vi "bangBangVelocityPlanning.vi"(0 "Game":refnum<class "Game.lvclass">, 5 "Robot in":refnum<class "Robot.lvclass">, 9 "Dest_array":T5(array[cluster]), 11 "type_of_use":T1, 12 "robots_test":T2[](array[typedef]), 13 "start":bool=TRUE) -> (4 "Robot out":refnum<class "Robot.lvclass">, 6 "replace":bool, 8 "velocityPlanningState":T3={"est_vel"=0.0, "dist_to_(Dest/L)"=0.0, "V0_model"=0.0, "max_dist_to_break"=0.0, "v_sent"=0.0, "traj_state"=enum."replace"})   [LabVIEW 2023, in "Game.lvclass"]
uses:
  Game.lvclass
  Robot_class/Robot.lvclass
  C:/Users/lucio/Desktop/roboime/SSL_AI/Object_class/Object.lvclass
  VelocityPlanningTest/Controls/velocityPlanningState.ctl
  VelocityPlanningTest/Controls/trajectoryState.ctl
  Communication_class/Paths/grSim Packet Command UDP Test Folder/grSim/grSim RobotReplacement.ctl
  Controls/typeOfUse.ctl
  Team_class/KeeperPlay.ctl
  Team_class/OffensivePlay.ctl
  Robot_class/Robot.lvclass/Robot.ctl
  Object_class/Object.lvclass/Object.ctl
  Game.lvclass/Game.ctl
  Team_class/Team.lvclass/Team.ctl
  Parameters_class/Parameters.lvclass/Parameters.ctl
  Robot_class/Read path_smooth.vi
  Object_class/Read x.vi
  Object_class/Read y.vi
  Robot_class/Write v_tang.vi
  Robot_class/Write v_norm.vi
  Robot_class/Write v_ang.vi
  Robot_class/Write est_v_norm.vi
  Robot_class/Write est_v_tang.vi
  <vilib>/Analysis/_algsub.llb/Real Vector Norm.vi
  Robot_class/Read orientation.vi
  Read OffensiveTeam.vi
  Read FieldRef.vi
  Read KeeperTeam.vi
  Read NewParameters.vi
  Read Parameters.lvclass.vi
  Parameters_class/Read PID gains Vel_desired.vi
  Parameters_class/Read StopVelocity.vi
  Parameters_class/Read Debug.vi
  Parameters_class/Read PID gains Angle.vi
  Parameters_class/Read PID gains Angle To Turn.vi
  Parameters_class/Read MaxOutputAngle.vi
  Parameters_class/Read bangBangParameters.vi
  Parameters_class/Read Enviroment.vi
  Parameters_class/Read PID per ID.vi
  Team_class/Read KeeperPlay.vi
  Team_class/Read OffensivePlay.vi
  Robot_class/Read robotKickState.vi
  Robot_class/Read dest_x.vi
  Robot_class/Read dest_y.vi
  Robot_class/Read v_tang.vi
  Robot_class/Read v_norm.vi
  Object_class/Read position(x,y).vi
  Ally_class/Ally.lvclass
  C:/Users/lucio/Desktop/roboime/SSL_AI/Team_class/Team.lvclass
  Field_class/Field.lvclass
  Parameters_class/Parameters.lvclass
  Utilities_class/Utilities.lvclass
  <vilib>/Analysis/NI_AALPro.lvlib
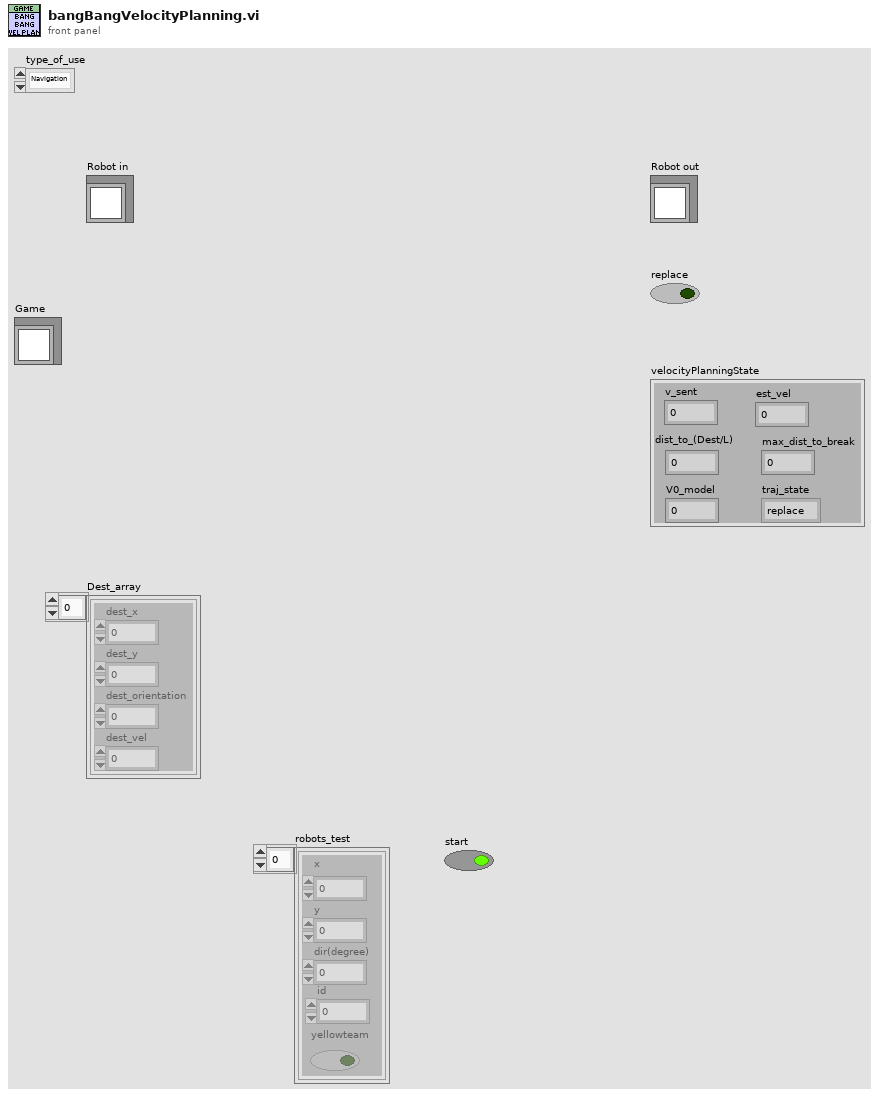
[diagram p1: front panel]
types:
  T1 = typedef "typeOfUse.ctl" = enum16{"Navigation", "ZigZag", "grSimTest"}
  T2 = typedef "grSim RobotReplacement.ctl" = cluster{"x":dbl, "y":dbl, "dir(degree)":dbl, "yellowteam":bool, "id":u32}
  T3 = typedef "velocityPlanningState.ctl" = cluster{"est_vel":dbl, "dist_to_(Dest/L)":dbl, "V0_model":dbl, "max_dist_to_break":dbl, "v_sent":dbl, "traj_state":T4}
  T4 = typedef "trajectoryState.ctl" = enum16{"stop", "replace", "circle", "line"}
  T5 = cluster{"dest_x":dbl, "dest_y":dbl, "dest_orientation":dbl, "dest_vel":dbl}[]
  T6 = typedef "OffensivePlay.ctl" = enum16{"5RobotsPassGamePlay", "5PreparePassGame", "5RobotsKeeperGame", "KeeperPassToStriker", "5RobotsNormalGamePlay", "PrepareKeeperPass", "ACBPass", "ABCPass", "PrepareTriplePass", "TableWithStriker", "TableWith2ndStrikerPlay", "PrepareDoublePass", "PrepareRollToPass", "SimplePass", "PreparePass", "PassToStriker", "BallOutOfField", "PassTo2ndStriker", "StopOffensive", "Prepare Penalty Enemy", "EnemyPossessionAtEnemyField", "EnemyPossesionAtOurField", "TestPlay", "PreparePenaltyAlly", "KickPenaltyAlly", "PrepareKickoffAlly", "PrepareKickoffEnemy", "IndirectEnemy", "DirectEnemy", "PreparePassInGame1", "NormalGame", "DirectKick", "Pass", "Halt", "Timeout", "PassPlay", "PenaltyEnemy"}
  T7 = typedef "KeeperPlay.ctl" = enum16{"SimpleBallPlacementAlly", "BallPlacementAlly", "BallPlacementEnemy", "ZigZag", "Goto", "NormalGame", "KeeperPlay", "Halt", "Timeout", "PenaltyEnemy", "TestPlay"}
  T8 = typedef "NewParameters.ctl" = cluster{"PenaltyDistance":dbl, "DistanceAttackerToBackBall":dbl, "Division":enum16{"Div B", "Div A"}, "DistanceToAvoidyEnemyRobot":dbl, "BallPlacementDistance":dbl, "DisatanceBehindBallToStealBall":dbl, "MaxDistanceToPositionKickoff":dbl, "BlockEnemyTarget":bool, "MaxStopVAng":dbl, "DistanceMarkerToEnemy":dbl, "IgnoreDribblerContact":bool, "DistanceToBeginEnemyPosession":dbl, "GoToBallWhenEnemyNotMoving":bool, "EnemyDistanceToReduceVelocity":dbl, "TurnOnEnemyDistanceToReduceVelocity":bool, "EnemyDistanceToShootOutBall":dbl, "DefenseKickBall":bool, "MoreKickToGoal? (0-0.3)":dbl, "ChipKickInEnemyField":bool, "ShootOutRobotId":dbl, "FieldLenghtDenominatorInShootOut":dbl, "AdjustPositionInBallPlacement":bool, "PowerGodPass":dbl, "VelocityAbortEnemyPos":dbl, "MaxDistToBeginPass":dbl, "MinDistToBeginPass":dbl, "VelocityInDirects":dbl, "BadDribblerIDs":i32[], "NewKickToDistanceAroundBall":dbl, "PowerAvoidColisionMarker":dbl, "DistanceToAvoidColisionMarker":dbl, "AvoidBallKick":dbl, "DistanceTryKick":dbl, "SuicideKickDIstance":dbl, "AdjustFirstKickDistance":dbl, "AvoidAimLessKick":dbl, "DistanceToAvoidyEnemyShootRobot ":dbl, "NumberOfMarkers":dbl, "PotField":bool, "PIDLateral":bool, "MinDistanceFirstKickX":dbl, "MinDistanceFirstKickY":dbl, "FractionOfDistToTouchGround\nAfterChipKick":dbl, "FractionOfKickxWhen\nComposedWithKickz":dbl, "Style":T9, "MoveInTurnState":bool, "DistFromEnemyToConsider\nMoveInTurnState":dbl, "CascadePID":bool, "TurnAroundParameters":cluster{"Radius":dbl, "Multiplier":dbl, "ChordAngle":dbl}, "SafeDriveVel":dbl, "DistanceToGoToBackBall":dbl, "minDistanceToNotFinishEnemyPossession":dbl, "OneTouchShot":cluster{"angleFactor":dbl, "maxAngle":dbl, "Attack":bool, "Defense":bool}, "OpenAngleToGoal":cluster{"minAngle":dbl, "maxAngle":dbl, "minEvaluation":dbl}, "ShotInterception":cluster{"shotSpeed":dbl, "minEnemySpeed":dbl, "maxEnemySpeed":dbl, "minEvaluation":dbl}, "AllyTeamArray":T10[], "maxDefendersNumber":i32, "Zone":cluster{"GuardPositionArray":dbl[][], "ZoneMidField":dbl[], "CenterForwardWidth":dbl}, "MinEvaluationToShoot":dbl, "PassInterception":cluster{"maxPassSpeed":dbl, "minPassSpeed":dbl, "minEnemySpeed":dbl, "chipPassDistance":dbl, "chipPassEvaluation":dbl, "minEvaluation":dbl, "maxEnemySpeed":dbl}, "PassDistance":cluster{"maxDistance":dbl, "minDistance":dbl}, "receiverSpeed":dbl, "maxBallSpeed":dbl, "slackTime":dbl}
  T9 = typedef "Style.ctl" = enum16{"Insanity", "Offensive", "Defensive"}
  T10 = typedef "AllyTeam.ctl" = enum16{"Keeper", "Defender", "Attacker"}
  T11 = cluster{"(Kc)":dbl, "(Ti, min)":dbl, "(Td, min)":dbl}
  T12 = typedef "bangBangControlParameters.ctl" = cluster{"MaxVSent":dbl, "MaxVNorm":dbl, "MaxVAng":dbl, "VAngCircle":dbl, "LBeginCircle":dbl, "DistToDestOrientation":dbl, "MaxVAngToTurn":dbl, "AtkDistToDestOrientation":dbl, "KepperMaxVSent":dbl, "VelNearEnemy":dbl}
  T13 = typedef "Enviroment.ctl" = enum16{"erForceSimulator", "grSim", "realGame"}
  T14 = typedef "robotKickToStates.ctl" = enum16{"shootFromDirect", "avoidCollideBall", "goToBackBall", "none", "walk", "turn", "oldKickToShoot", "oldKickToGoToBackBall", "shoot"}
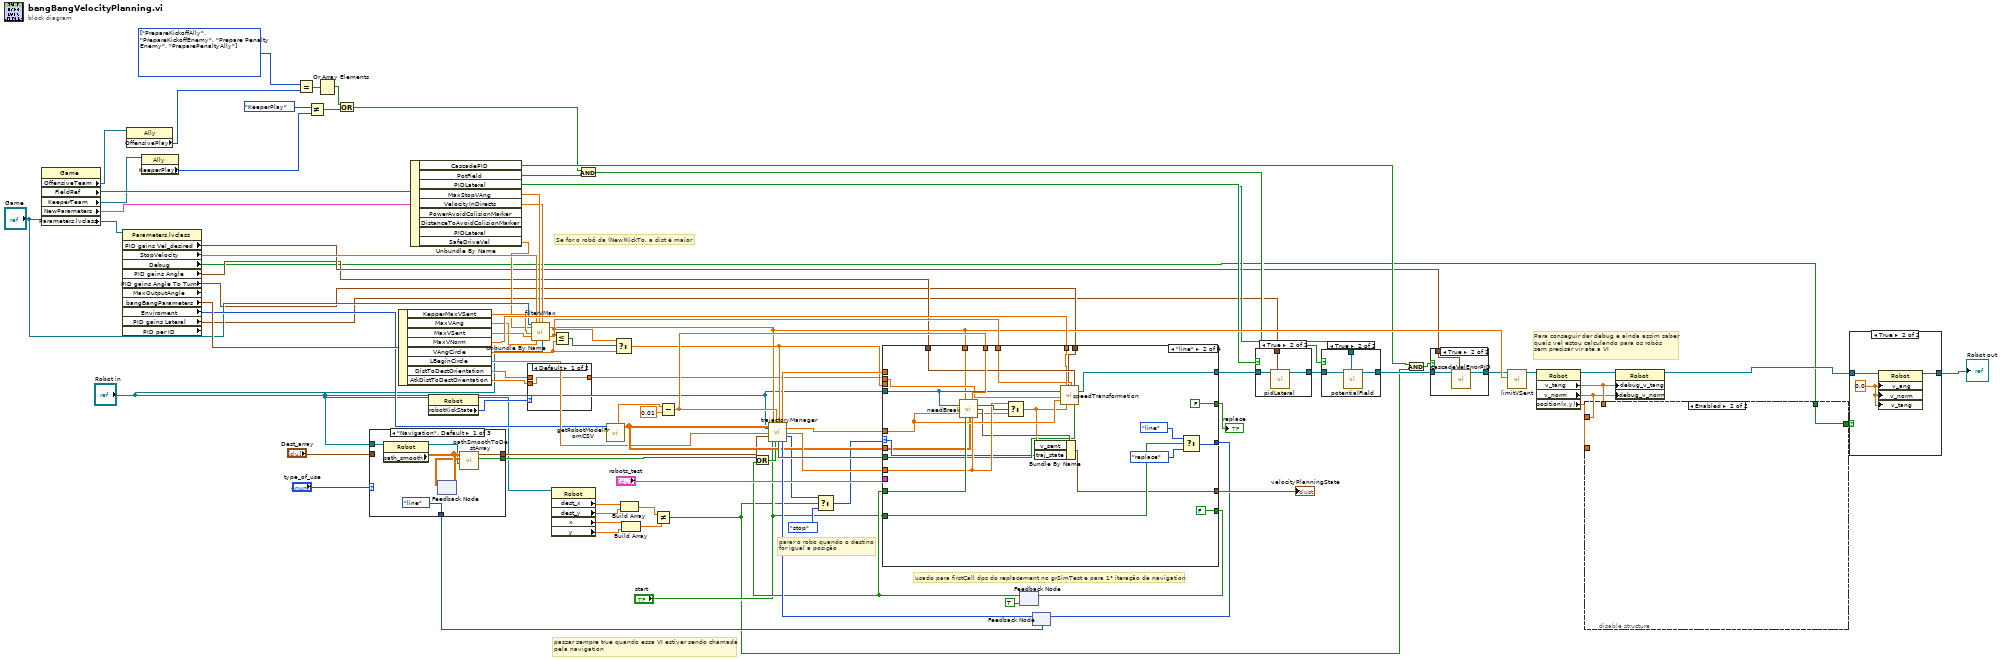
[diagram p0: block diagram]
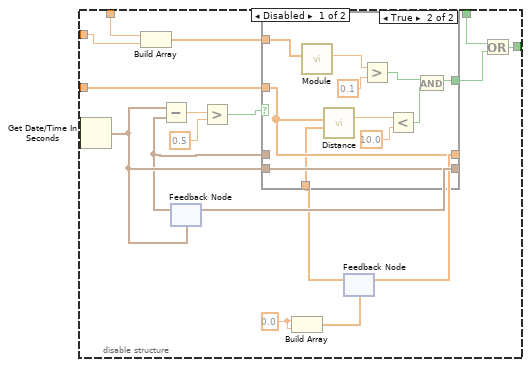
[diagram p2: hidden frame]
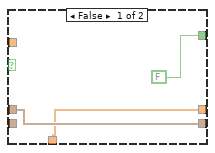
[diagram p3: hidden frame]
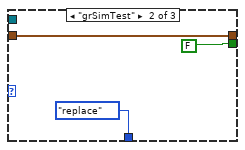
[diagram p8: hidden frame]
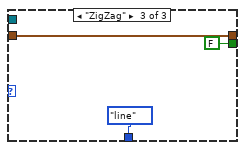
[diagram p9: hidden frame]
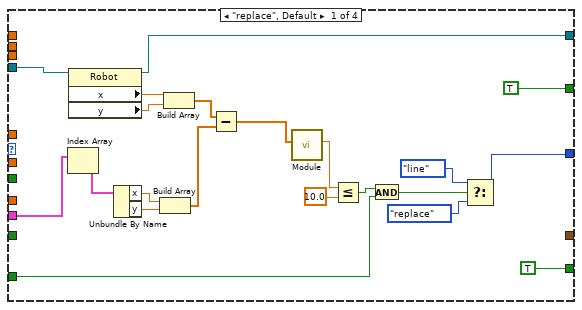
[diagram p10: hidden frame]
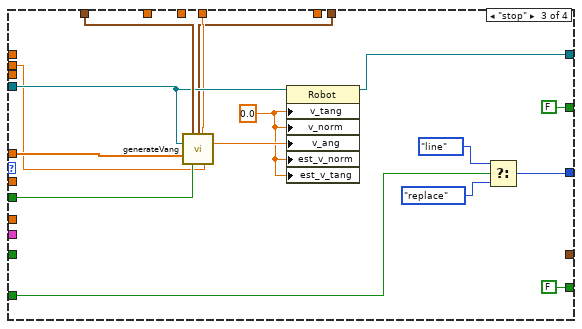
[diagram p11: hidden frame]
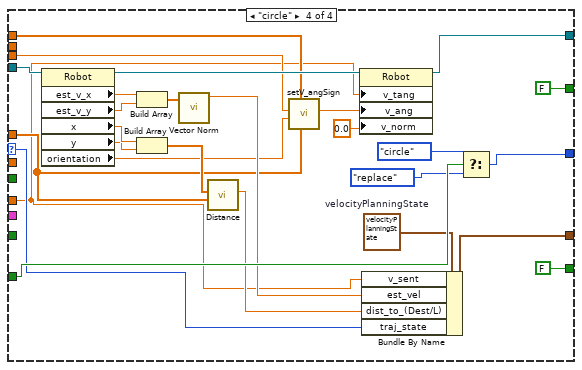
[diagram p12: hidden frame]
diagram:
  w16 = T6[] [enum."PrepareKickoffAlly", enum."PrepareKickoffEnemy", enum."Prepare Penalty Enemy", enum."PreparePenaltyAlly"] items=["5RobotsPassGamePlay", "5PreparePassGame", "5RobotsKeeperGame", "KeeperPassToStriker", "5RobotsNormalGamePlay", "PrepareKeeperPass", "ACBPass", "ABCPass", "PrepareTriplePass", "TableWithStriker", "TableWith2ndStrikerPlay", "PrepareDoublePass", "PrepareRollToPass", "SimplePass", "PreparePass", "PassToStriker", "BallOutOfField", "PassTo2ndStriker", "StopOffensive", "Prepare Penalty Enemy", "EnemyPossessionAtEnemyField", "EnemyPossesionAtOurField", "TestPlay", "PreparePenaltyAlly", "KickPenaltyAlly", "PrepareKickoffAlly", "PrepareKickoffEnemy", "IndirectEnemy", "DirectEnemy", "PreparePassInGame1", "NormalGame", "DirectKick", "Pass", "Halt", "Timeout", "PassPlay", "PenaltyEnemy"] ("x")
  # "parar o robo quando o destino\nfor igual a posição"
  # "Para conseguir dar debug e ainda assim saber\nquais vel estou calculando para os robôs\nsem precisar vir até a VI"
  # "Se for o robô da (New)KickTo, a dist é maior"
  # "usado para firstCall dps do replacement no grSimTest e para 1° iteração da navigation"
  # "passar sempre true quando essa VI estiver sendo chamada\npela navigation"
  n1 = property class="Game" props=["OffensiveTeam", "FieldRef", "KeeperTeam", "NewParameters", "Parameters.lvclass"](reference="Game") -> (reference out=w41:refnum<class "Game.lvclass">, "OffensiveTeam"=w17:refnum<class "Ally.lvclass">, "KeeperTeam"=w21:refnum<class "Ally.lvclass">, "NewParameters"=w54:T8, "Parameters.lvclass"=w61:refnum<class "Parameters.lvclass">)  [unwired: 1 in, 2 out]
  n2 = property class="Parameters.lvclass" props=["PID gains Vel_desired", "StopVelocity", "Debug", "PID gains Angle", "PID gains Angle To Turn", "MaxOutputAngle", "bangBangParameters", "Enviroment", "PID gains Lateral", "PID per ID"](reference=w61) -> ("PID gains Vel_desired"=w10:T11, "StopVelocity"=w59:dbl, "Debug"=w4:bool, "PID gains Angle"=w9:cluster{"(Kc)":dbl, "(Ki)":dbl, "(Kd)":dbl}, "PID gains Angle To Turn"=w8:cluster{"(Kc)":dbl, "(Ki)":dbl, "(Kd)":dbl}, "bangBangParameters"=w66:T12, "Enviroment"=w62:T13, "PID gains Lateral"=w7:cluster{"(Kc)":dbl, "(Ki)":dbl, "(Kd)":dbl})  [unwired: 1 in, 4 out]
  n3 = property class="Ally"(reference=w17) -> ("OffensivePlay"=w11:T6)  [unwired: 1 in, 2 out]
  n4 = property class="Ally"(reference=w21) -> ("KeeperPlay"=w20:T7)  [unwired: 1 in, 2 out]
  n5 = Equal?(x=w16, y=w11) -> (x = y?=w15:bool[])
  n6 = Not Equal?(x=KeeperPlay."KeeperPlay", y=w20) -> (x != y?=w13:bool)
  n7 = Or Array Elements(Boolean array=w15) -> (logical OR=w14:bool)
  n8 = Or(x=w14, y=w13) -> (x .or. y?=w12:bool)
  n9 = case shown="\"Navigation\", Default" "type_of_use" {
    tunnel: "Robot in" -> [w98 _ _]
    tunnel: [w95 w101 w104] -> w74
    tunnel: [w94 FALSE FALSE ("new_path_smooth?")] -> w73
    tunnel: "Dest_array" -> [_ w101 w104]
    tunnel: [trajectoryState."line" ("traj_state out") trajectoryState."replace" ("traj_state out") trajectoryState."line" ("traj_state out")] -> w69
    frame "Navigation", Default {
      n10 = property class="Robot"(reference=w98) -> (reference out=w92:refnum<class "Robot.lvclass">, "path_smooth"=w97:dbl[][])  [unwired: 1 in, 1 out]
      n11 = feedback #1() -> (w96:dbl[][])  [unwired: 1 in]
      n12 = feedback-in #1(w97) -> ()
      n13 = call "pathSmoothToDestArray.vi"("Robot"=w92, "last_path_smooth"=w96, "path_smooth"=w97) -> ("new_path_smooth?"=w94:bool, "dest_array"=w95:T5)  [unwired: 7 in]
    }
    frame "grSimTest" {
    }
    frame "ZigZag" {
    }
  }
  n14 = Unbundle By Name(w66) -> ("KepperMaxVSent"=w50:dbl, "MaxVAng"=w53:dbl, "MaxVSent"=w60:dbl, "MaxVNorm"=w64:dbl, "VAngCircle"=w65:dbl, "LBeginCircle"=w63:dbl, "DistToDestOrientation"=w57:dbl, "AtkDistToDestOrientation"=w55:dbl)
  n15 = Unbundle By Name(w54) -> ("CascadePID"=w26:bool, "PotField"=w22:bool, "PIDLateral"=w44:bool, "MaxStopVAng"=w52:dbl, "VelocityInDirects"=w49:dbl, "SafeDriveVel"=w38:dbl)  [unwired: 3 out]
  n16 = property class="Robot"(reference="Robot in") -> (reference out=w37:refnum<class "Robot.lvclass">, "robotKickState"=w58:T14)  [unwired: 1 in, 1 out]
  n17 = case shown="Default" w58 {
    tunnel: [w105 w106] -> w56
    tunnel: w57 -> [_ w106]
    tunnel: w55 -> [w105 _]
    frame Default {
    }
    frame "none" {
    }
  }
  n18 = call "filterVMax.vi"("Game in"="Game", "safeDriveVel"=w38, "KepperMaxVSent"=w50, "MaxVSent"=w60, "StopVelocity"=w59, "MaxVAng"=w53, "MaxStopVAng"=w52, "VelocityInDirects"=w49, "Robot in"="Robot in") -> ("MaxVSent out"=w47:dbl, "MaxVAng out"=w51:dbl)  [unwired: 7 in, 2 out]
  n19 = property class="Robot"(reference=w37) -> ("dest_x"=w36:dbl, "dest_y"=w35:dbl, "x"=w33:dbl, "y"=w32:dbl)  [unwired: 1 in, 2 out]
  n20 = Less Or Equal?(x=w51, y=w65) -> (x <= y?=w68:bool)
  n21 = And(x=w12, y=w22) -> (x .and. y?=w18:bool)
  n22 = call "getRobotModelFromCSV.vi"("Environment"=w62) -> ("robotModel"=w79:dbl[][], "delta"=w77:dbl)  [unwired: 9 in]
  n23 = Select(t=w51, s=w68, f=w65) -> (s? t:f=w67:dbl)
  n24 = Build Array(w36, w35) -> (w34:dbl[])
  n25 = Build Array(w33, w32) -> (w31:dbl[])
  n26 = Not Equal?(x=w34, y=w31) -> (x != y?=w24:bool)
  n27 = Subtract(x=w77, y=0.01) -> (x-y=w76:dbl)
  n28 = feedback #2(TRUE) -> (w75:bool)
  n29 = Or(x=w73, y=w75) -> (x .or. y?=w72:bool)
  n30 = feedback #3(w69) -> (w87:T4)
  n31 = call "trajectoryManager.vi"("Robot"="Robot in", "robotModel"=w79, "L"=w63, "Dest_array"=w74, "max_v_sent"=w47, "start"="start", "delta"=w76, "firstCall"=w72, "v_ang_curve"=w67, "traj_state"=w87) -> ("last_dest"=w89:bool, "next_dest"=w90:dbl[], "Dest"=w85:dbl[], "v_desired"=w86:dbl, "traj_state out"=w29:T4)  [unwired: 3 in, 2 out]
  n32 = Select(t=w29, s=w24, f=trajectoryState."stop") -> (s? t:f=w30:T4)
  n33 = case shown="\"line\"" w30 {
    selector: w30 -> [_ w136 _ w172]
    tunnel: "Robot in" -> [w117 w145 w165 w196]
    tunnel: "robots_test" -> [w116 _ _ _]
    tunnel: [TRUE FALSE FALSE FALSE] -> w91
    tunnel: [w114 w150 w157 w187] -> w80
    tunnel: [w113 w143 w169 w194] -> w46
    tunnel: w85 -> [_ w144 w164 w174]
    tunnel: "start" -> [w110 w151 w156 w190]
    tunnel: [TRUE FALSE FALSE FALSE] -> w82
    tunnel: w75 -> [_ w148 _ _]
    tunnel: [_ w140 _ w186] -> w84
    tunnel: w76 -> [_ w147 _ _]
    tunnel: w86 -> [_ w146 _ w171]
    tunnel: w89 -> [_ w137 w163 _]
    tunnel: w90 -> [_ _ _ w176]
    tunnel: w67 -> [_ _ _ w175]
    tunnel: w47 -> [_ w129 _ _]
    tunnel: w79 -> [_ w135 _ _]
    tunnel: w9 -> [_ w134 w166 _]
    tunnel: w51 -> [_ w132 w162 _]
    tunnel: w64 -> [_ w133 _ _]
    tunnel: w56 -> [_ w131 w160 _]
    tunnel: w8 -> [_ w130 w155 _]
    frame "replace", Default {
      n34 = Index Array(array=w116) -> (element=w124:T2)  [unwired: 1 in]
      n35 = property class="Robot"(reference=w117) -> (reference out=w113:refnum<class "Robot.lvclass">, "x"=w127:dbl, "y"=w126:dbl)  [unwired: 1 in, 1 out]
      n36 = Unbundle By Name(w124) -> ("x"=w123:dbl, "y"=w122:dbl)
      n37 = Build Array(w123, w122) -> (w121:dbl[])
      n38 = Build Array(w127, w126) -> (w125:dbl[])
      n39 = Subtract(x=w125, y=w121) -> (x-y=w120:dbl[])
      n40 = call "Module.vi"("2D vector"=w120) -> ("Modulo"=w119:dbl)  [unwired: 8 in, 2 out]
      n41 = Less Or Equal?(x=w119, y=10.0) -> (x <= y?=w111:bool)
      n42 = And(x=w111, y=w110) -> (x .and. y?=w112:bool)
      n43 = Select(t=trajectoryState."line" ("traj_state out"), s=w112, f=trajectoryState."replace" ("traj_state out")) -> (s? t:f=w114:T4)
    }
    frame "line" {
      n44 = call "needBreak.vi"("v_sample"=w129, "delta"=w147, "Robot"=w145, "dest"=w144, "firstCall"=w148, "robotModel"=w135, "desired_vel"=w146) -> ("needBreak"=w152:bool, "velocityPlanningState"=w142:T3, "vel"=w128:dbl)  [unwired: 4 in, 2 out]
      n45 = Select(t=w146, s=w152, f=w128) -> (s? t:f=w141:dbl)
      n46 = Bundle By Name(cluster=w142, "v_sent"=w141, "traj_state"=w136) -> (w140:T3)
      n47 = call "speedTransformation.vi"("Robot"=w145, "DistToDestOrientation"=w131, "Dest"=w144, "V_norm_limit"=w133, "V_sent"=w141, "PID Gains Angle To Turn"=w130, "Vang_limit"=w132, "PID Gains Angle"=w134, "last_dest"=w137) -> ("Robot out"=w143:refnum<class "Robot.lvclass">)  [unwired: 8 in, 2 out]
      n48 = Select(t=trajectoryState."line" ("traj_state out"), s=w151, f=trajectoryState."replace" ("traj_state out")) -> (s? t:f=w150:T4)
    }
    frame "stop" {
      w154 = 0.0 ("v_ang")
      n49 = call "generateVang.vi"("PID Gains Angle"=w166, "PID Gains Angle To Turn"=w155, "Vang_limit"=w162, "Robot"=w165, "Dest"=w164, "last_dest"=w163, "DistToDestOrientation"=w160) -> ("Vang"=w161:dbl)  [unwired: 6 in, 2 out]
      n50 = property class="Robot"(reference=w165, "v_tang"=w154, "v_norm"=w154, "v_ang"=w161, "est_v_norm"=w154, "est_v_tang"=w154) -> (reference out=w169:refnum<class "Robot.lvclass">)  [unwired: 1 in, 1 out]
      n51 = Select(t=trajectoryState."line" ("traj_state out"), s=w156, f=trajectoryState."replace" ("traj_state out")) -> (s? t:f=w157:T4)
    }
    frame "circle" {
      w170 = T3 {"est_vel"=0.0, "dist_to_(Dest/L)"=0.0, "V0_model"=0.0, "max_dist_to_break"=0.0, "v_sent"=0.0, "traj_state"=enum."replace"}  # velocityPlanningState
      n52 = property class="Robot"(reference=w196) -> (reference out=w195:refnum<class "Robot.lvclass">, "est_v_x"=w185:dbl, "est_v_y"=w184:dbl, "x"=w181:dbl, "y"=w180:dbl, "orientation"=w173:dbl)  [unwired: 1 in, 1 out]
      n53 = Build Array(w185, w184) -> (w183:dbl[])
      n54 = Build Array(w181, w180) -> (w179:dbl[])
      n55 = call-poly <vilib>:"Vector Norm.vi"("Input Vector"=w183) -> ("norm"=w182:dbl)  [unwired: 9 in, 1 out]
      n56 = call "Distance.vi"("P1"=w174, "P2"=w179) -> ("Distance"=w178:dbl)  [unwired: 7 in, 2 out]
      n57 = call "setV_angSign.vi"("current_dest"=w174, "next_dest"=w176, "orientation"=w173, "v_ang"=w175) -> ("v_ang_with_sign"=w177:dbl)  [unwired: 5 in, 2 out]
      n58 = property class="Robot"(reference=w195, "v_tang"=w171, "v_ang"=w177, "v_norm"=0.0) -> (reference out=w194:refnum<class "Robot.lvclass">)  [unwired: 1 in, 1 out]
      n59 = Bundle By Name(cluster=w170, "v_sent"=w171, "est_vel"=w182, "dist_to_(Dest/L)"=w178, "traj_state"=w172) -> (w186:T3)
      n60 = Select(t=trajectoryState."circle" ("traj_state out"), s=w190, f=trajectoryState."replace" ("traj_state out")) -> (s? t:f=w187:T4)
    }
  }
  "replace" <- w91
  "velocityPlanningState" <- w84
  n61 = feedback-in #2(w82) -> ()
  n62 = feedback-in #3(w80) -> ()
  n63 = case shown="True" w44 {
    tunnel: w46 -> [w197 w200]
    tunnel: [w197 w199] -> w45
    tunnel: w7 -> [_ w198]
    frame False {
    }
    frame True {
      n64 = call "pidLateral.vi"("PID gains Lateral"=w198, "Robot in"=w200) -> ("Robot out"=w199:refnum<class "Robot.lvclass">)  [unwired: 8 in, 1 out]
    }
  }
  n65 = case shown="True" w18 {
    tunnel: [w201 w204] -> w40
    tunnel: w41 -> [_ w203]
    tunnel: w45 -> [w201 w202]
    frame False {
    }
    frame True {
      n66 = call "potentialField.vi"("Game"=w203, "Robot in"=w202) -> ("Robot out"=w204:refnum<class "Robot.lvclass">)  [unwired: 8 in, 1 out]
    }
  }
  n67 = And(x=w26, y=w24) -> (x .and. y?=w25:bool)
  n68 = case shown="True" w25 {
    tunnel: w10 -> [_ w206]
    tunnel: w40 -> [w205 w208]
    tunnel: [w205 w207] -> w39
    frame False {
    }
    frame True {
      n69 = call "cascadeVelErrorPID.vi"("PID gains"=w206, "Robot in"=w208) -> ("Robot out"=w207:refnum<class "Robot.lvclass">)  [unwired: 8 in, 1 out]
    }
  }
  n70 = call "limitVSent.vi"("MaxVSent"=w47, "Robot in"=w39) -> ("Robot out"=w43:refnum<class "Robot.lvclass">)  [unwired: 9 in]
  n71 = property class="Robot"(reference=w43) -> (reference out=w42:refnum<class "Robot.lvclass">, "v_tang"=w2:dbl, "v_norm"=w1:dbl, "position(x,y)"=w5:dbl[])  [unwired: 1 in, 1 out]
  n72 = disable-structure shown="Enabled" {
    disable-tunnel: w5 -> [w215 _]
    disable-tunnel: w4 -> [w214 w240]
    disable-tunnel: [w213 w240] -> w3
    disable-tunnel: w2 -> [w211 _]
    disable-tunnel: w1 -> [w210 _]
    frame Disabled {
      w219 = 0.0 ("element")
      n73 = Get Date/Time In Seconds() -> (seconds since 1Jan1904=w222:timestamp)
      n74 = Build Array(w211, w210) -> (w209:dbl[])
      n75 = feedback #4(w222) -> (w220:timestamp)
      n76 = Subtract(x=w222, y=w220) -> (x-y=w225:dbl)
      n77 = Greater?(x=w225, y=0.5) -> (0:w223:bool)
      n78 = Build Array(w219, w219) -> (w218:dbl[])
      n79 = feedback #5(w218) -> (w217:dbl[])
      n80 = case shown="True" w223 {
        tunnel: w222 -> [_ w239]
        tunnel: [w228 w239] -> w221
        tunnel: w220 -> [w228 _]
        tunnel: w217 -> [w227 w237]
        tunnel: [w227 w238] -> w216
        tunnel: w215 -> [_ w238]
        tunnel: [FALSE w233] -> w212
        tunnel: w209 -> [_ w232]
        frame False {
        }
        frame True {
          n81 = call "Module.vi"("2D vector"=w232) -> ("Modulo"=w231:dbl)  [unwired: 8 in, 2 out]
          n82 = call "Distance.vi"("P1"=w237, "P2"=w238) -> ("Distance"=w236:dbl)  [unwired: 7 in, 2 out]
          n83 = Greater?(x=w231, y=0.1) -> (0:w229:bool)
          n84 = Less?(x=w236, y=10.0 ("Distance")) -> (x < y?=w234:bool)
          n85 = And(x=w229, y=w234) -> (x .and. y?=w233:bool)
        }
      }
      n86 = feedback-in #4(w221) -> ()
      n87 = feedback-in #5(w216) -> ()
      n88 = Or(x=w214, y=w212) -> (x .or. y?=w213:bool)
    }
    frame Enabled {
    }
  }
  n89 = property class="Robot"(reference=w42, "debug_v_tang"=w2, "debug_v_norm"=w1) -> (reference out=w6:refnum<class "Robot.lvclass">)  [unwired: 1 in, 1 out]
  n90 = case shown="True" w3 {
    tunnel: [w241 w244] -> w88
    tunnel: w6 -> [w241 w243]
    frame False {
    }
    frame True {
      w242 = 0.0 ("v_ang")
      n91 = property class="Robot"(reference=w243, "v_ang"=w242, "v_norm"=w242, "v_tang"=w242) -> (reference out=w244:refnum<class "Robot.lvclass">)  [unwired: 1 in, 1 out]
    }
  }
  "Robot out" <- w88
